vi "Device.Init.vi"(8 "error in (no error)":errorcluster, 11 "MC.DangwooOptron in":refnum<class "MC.DangwooOptron.lvclass">) -> (0 "error out":errorcluster, 2 "Result":bool, 3 "MC.DangwooOptron out":refnum<class "MC.DangwooOptron.lvclass">)   [LabVIEW 2017, in "MC.DangwooOptron.lvclass"]
uses:
  MC.DangwooOptron.lvclass
  D:/upwork/Laser Measurement Tool/Laser/project/Subsystems/MC/MC/MC.lvclass
  Typedefs/Resource--Cluster.ctl
  <vilib>/Instr/_visa.llb/VISA Configure Serial Port (Instr).vi
  MC/MC.lvclass
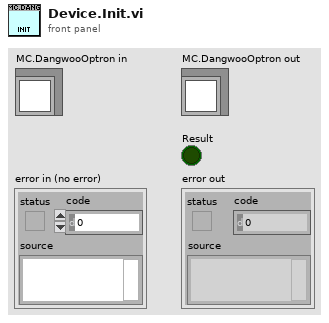
[diagram p1: front panel]
types:
  T1 = typedef "MC.DangwooOptron.lvclass/Resource--Cluster.ctl" = cluster{"VISA resource":refnum<visa-resource-name>}
  T2 = typedef "MC.lvclass/Configuration--Cluster.ctl" = cluster{"VISA Resource":string}
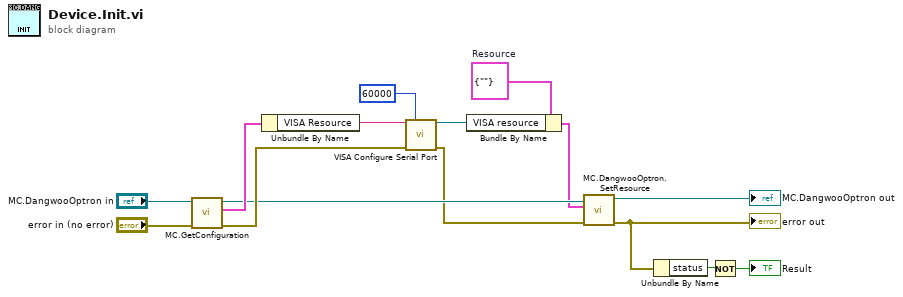
[diagram p0: block diagram]
diagram:
  w9 = T1 {"VISA resource"=""}  # Resource
  n1 = call "MC.GetConfiguration.vi"("error in (no error)"="error in (no error)", "MC"="MC.DangwooOptron in") -> ("error out"=w11:errorcluster, "Configuration"=w13:T2, "MC out"=w7:refnum<class "MC.DangwooOptron.lvclass">)  [unwired: 7 in]
  n2 = Unbundle By Name(w13) -> ("VISA Resource"=w12:string)
  n3 = call-poly "VISA Configure Serial Port"("VISA resource name"=w12, "timeout (10sec)"=u32 60000, "error in (no error)"=w11) -> ("VISA resource name out"=w8:refnum<visa-resource-name>, "error out"=w6:errorcluster)  [unwired: 11 in]
  n4 = Bundle By Name(cluster=w9, "VISA resource"=w8) -> (w5:T1)
  n5 = call "MC.DangwooOptron.SetResource.vi"("error in (no error)"=w6, "Resource"=w5, "MC.DangwooOptron"=w7) -> ("error out"=w1:errorcluster, "MC.DangwooOptron out"=→"MC.DangwooOptron out":refnum<class "MC.DangwooOptron.lvclass">)  [unwired: 7 in]
  "error out" <- w1
  n6 = Unbundle By Name(w1) -> ("status"=w4:bool)
  n7 = Not(x=w4) -> (.not. x?=→"Result":bool)
